vi "001 Llegir els valors d’un Cluster.vi"() -> ()   [LabVIEW 2019]
panel:
  out "Telèfon":string
  out "Adreça":string
  out "Nom  i cognoms":string
  in  "Cluster prova":T1
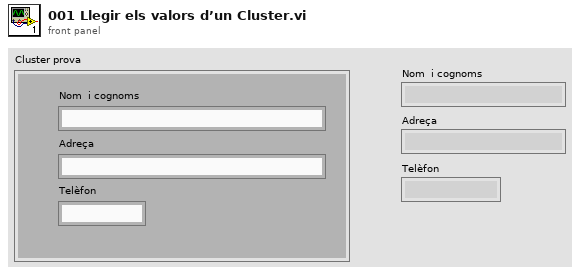
[diagram p1: front panel]
types:
  T1 = cluster{"Nom  i cognoms":string, "Adreça":string, "Telèfon":string}
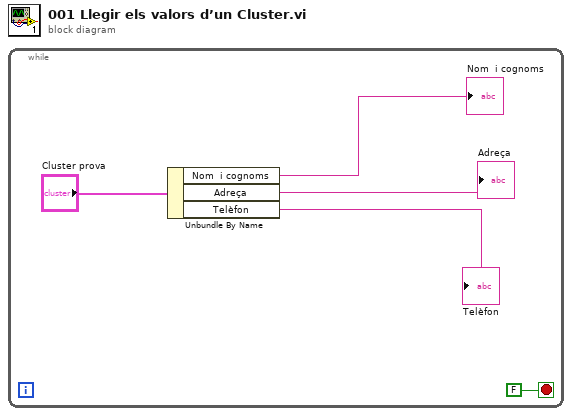
[diagram p0: block diagram]
diagram:
  n1 = while {
    stop <- FALSE stop-if-true
    n2 = Unbundle By Name("Cluster prova") -> ("Nom  i cognoms"=→"Nom  i cognoms":string, "Adreça"=→"Adreça":string, "Telèfon"=→"Telèfon":string)
  }
